vi "Close.vi"(8 "error in":errorcluster, 11 "DAQmx Base Configure Strategy in":refnum<class "DAQmx Base Configure Strategy.lvclass">) -> (0 "error out":errorcluster, 3 "DAQmx Base Configure Strategy out":refnum<class "DAQmx Base Configure Strategy.lvclass">)   [LabVIEW 2024, in "DAQmx Base Configure Strategy.lvclass"]
uses:
  DAQmx Base Configure Strategy.lvclass
  DAQmx Base Configure Strategy.lvclass/DAQmx Base Configure Strategy.ctl
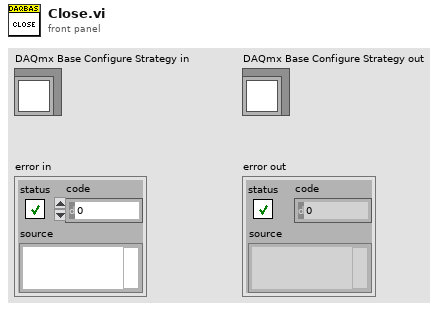
[diagram p1: front panel]
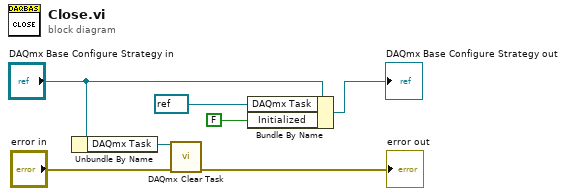
[diagram p0: block diagram]
diagram:
  n1 = Unbundle By Name("DAQmx Base Configure Strategy in") -> ("DAQmx Task"=w6:refnum<k21>)
  n2 = call <vilib>:"DAQmx Clear Task.vi"("task in"=w6, "error in"="error in") -> ("error out"=→"error out":errorcluster)  [unwired: 13 in]
  n3 = Bundle By Name(cluster="DAQmx Base Configure Strategy in", "DAQmx Task"=refnum<k21> refnum ("Task"), "Initialized"=FALSE) -> (→"DAQmx Base Configure Strategy out":refnum<class "DAQmx Base Configure Strategy.lvclass">)
